vi "LDA_Analysis_2.vi"() -> (5 "Plug in titles":string[](array[string]), 7 "Plug in values":string[](array[string]))   [LabVIEW 2010]
uses:
  Controls/Save_Data.ctl
  Globals/LDA_meas_global_1.vi
  Globals/Plug_in_data_global.vi
  Globals/Meas_global.vi
  Globals/Constants_global.vi
  <vilib>/Analysis/NI_AALBase.lvlib
panel:
  out "Uneven timetrace":cluster{"Freq":dbl[], dbl[]}(graph)
  out "XY Graph 2":cluster{"Freq":dbl[], dbl[]}[](graph)
  in  "No of estimates output":i32=300
  out "Autocorrelation":cluster{dbl, dbl, dbl[]}[](graph)
  in  "Mode":enum16{"Spectra", "Autocorrelation"}(ring)
  in  "Separation Character":string="\t"
  in  "Precision":i16=2
  out "Ch names":string[](array[string])
  out "Number or Good blocks":i32
  out "Resampled block length":i32
  out "Resampling Frequency":dbl
  in  "Output Directory":path
  in  "File":T1=enum."Save Data"
  out "Frequency Spectrum":cluster{dbl, dbl, dbl[]}[](graph)
  # "You must have just these two indicators on the connector pane of the vi"
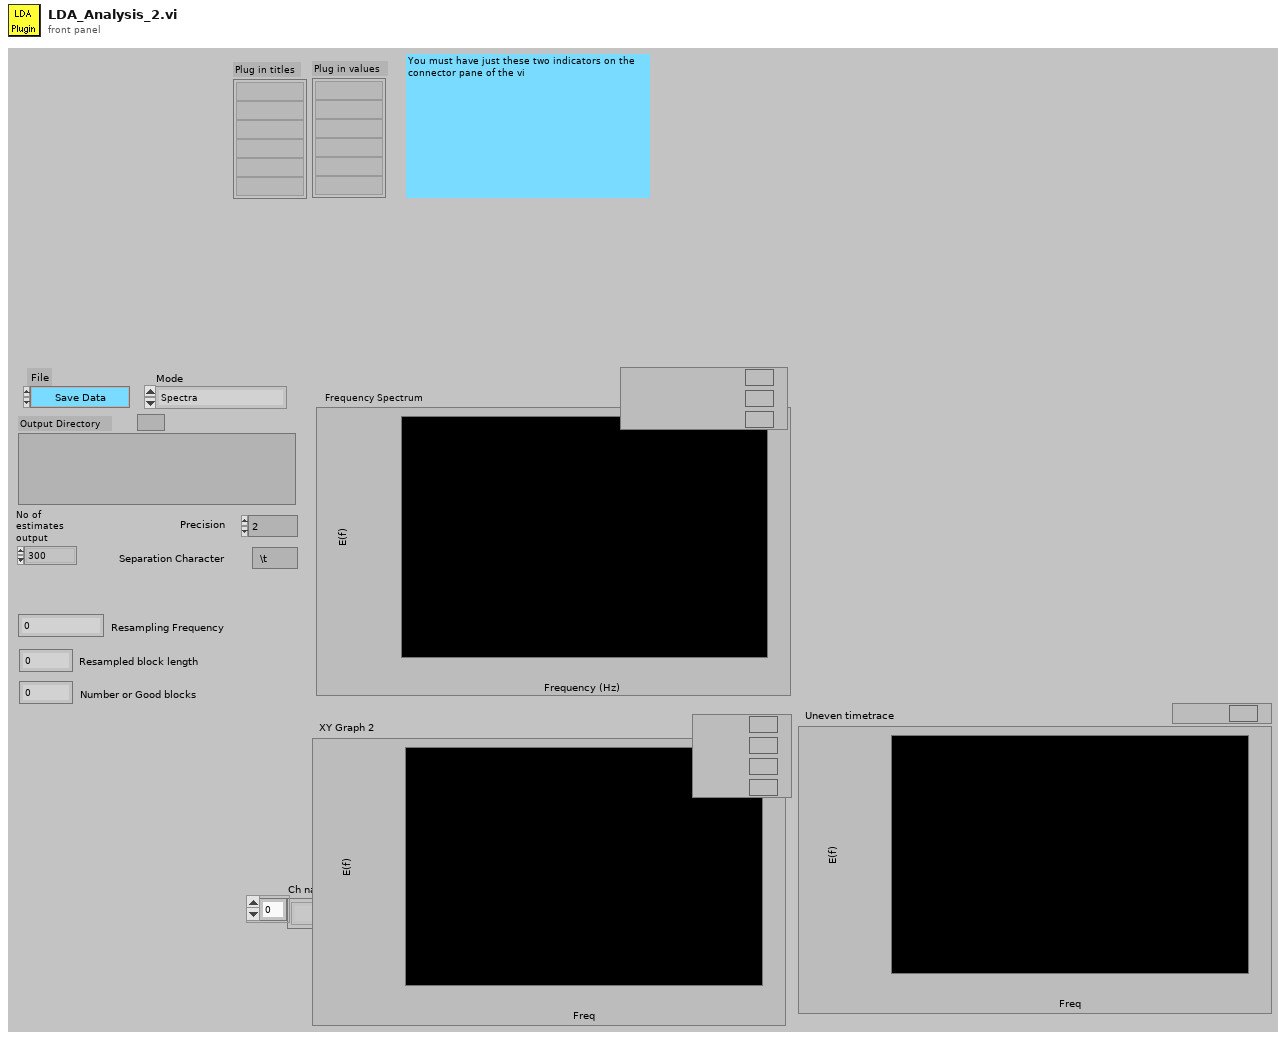
[diagram p1: front panel]
types:
  T1 = typedef "Save_Data.ctl" = enum16{"Save No Data", "Save Data"}
  T2 = enum32{"existing file", "new file", "new or existing file", "existing dir", "new dir", "new or existing dir", "existing file (use LLBs)", "new file (use LLBs)", "new or existing file (use LLBs)", "new or existing file or directory (use LLBs)"}
  T3 = typedef "Analysis_info_cluster.ctl" = cluster{"Colour":u32, "Inst type":T4, "Inst name":string, "Symbol":string, "Code name":string, "Extra Info":string, "Inst Array":T5, "Index":i32, "Voltage Index":i32, "Extra Titles":string[], "Extra Values":string[]}
  T4 = typedef "Inst_type.ctl" = enum16{"Propeller anemometer", "Raw voltage", "Pressure Transducer", "Pitot-static tube", "Preston tube", "Hot wire", "Cross wire 1", "Cross wire 2", "Generic Linear", "Generic Polynomial", "Generic BackPoly", "Fast FID", "Thermocouple", "Cold wire", "Pulsed Wire", "LDA Vel", "LDA Tran time", "LDA Arr time"}
  T5 = typedef "Instrument_Array.ctl" = enum16{"PWA", "LDA", "Analogue"}
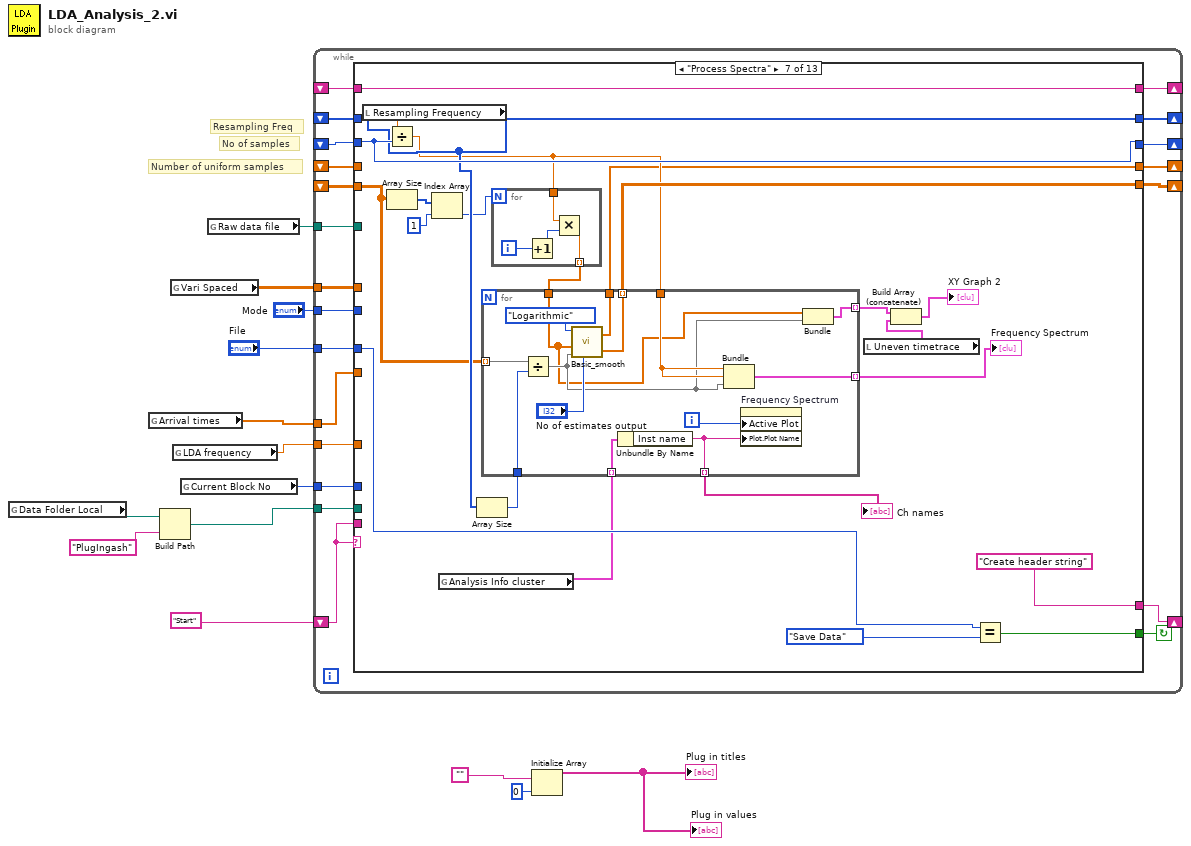
[diagram p0: block diagram]
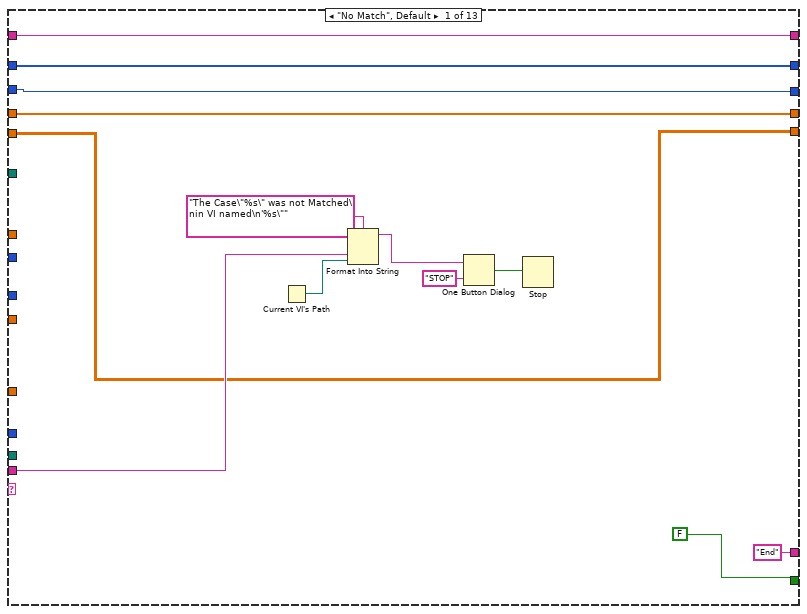
[diagram p2: hidden frame]
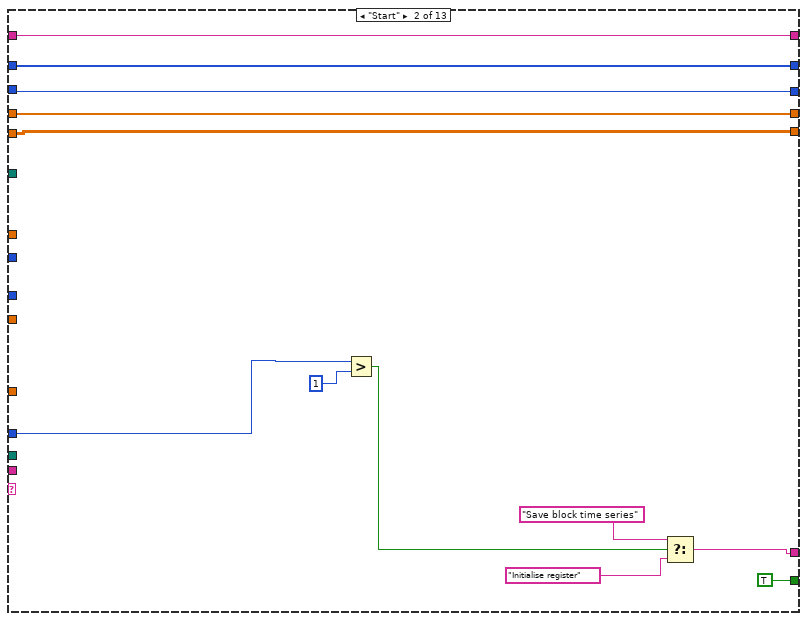
[diagram p3: hidden frame]
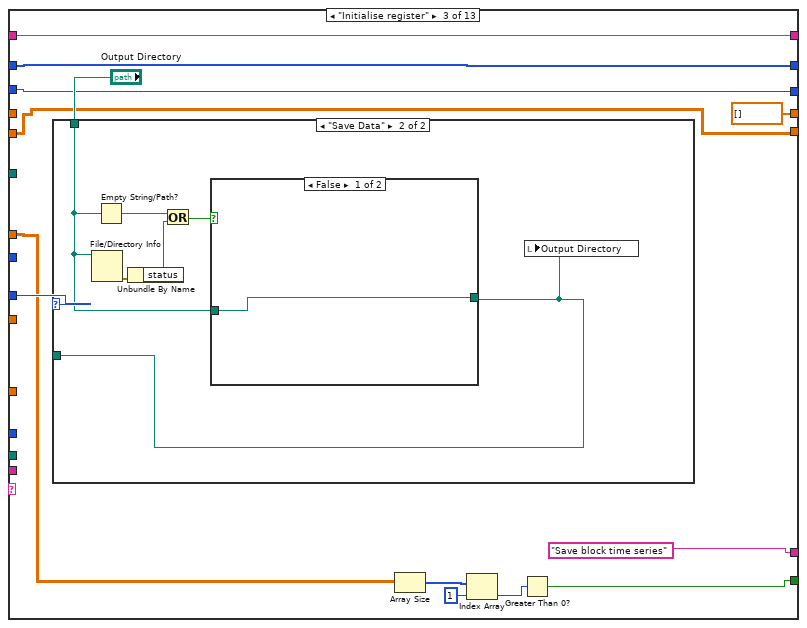
[diagram p4: hidden frame]
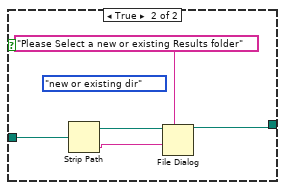
[diagram p6: hidden frame]
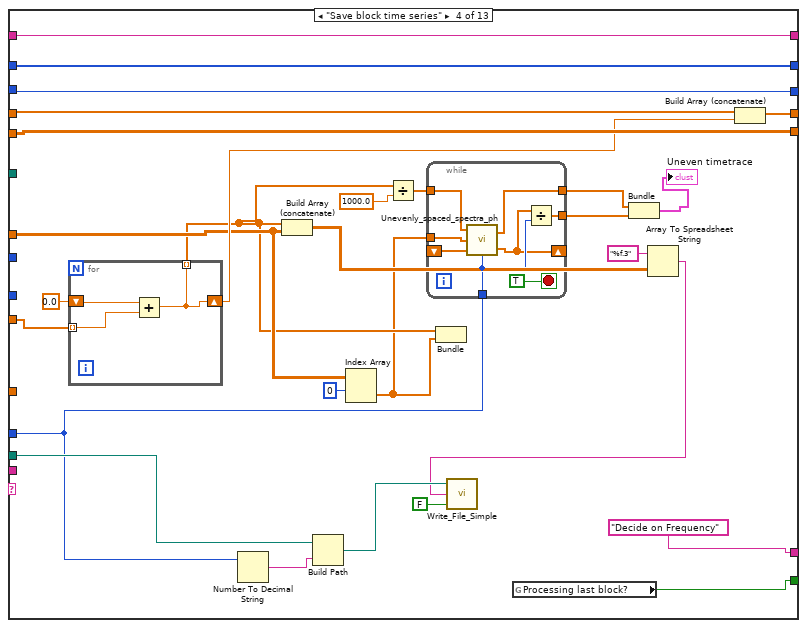
[diagram p7: hidden frame]
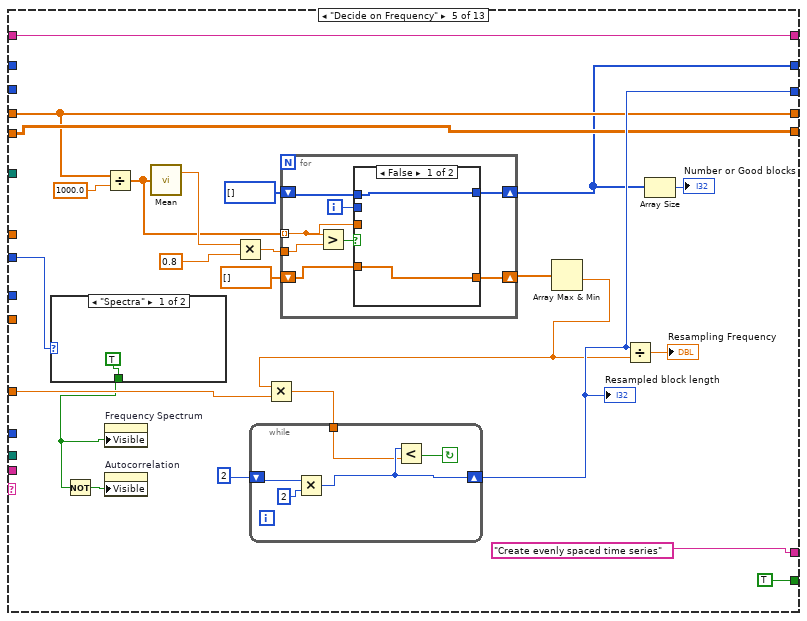
[diagram p8: hidden frame]
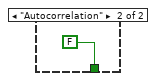
[diagram p9: hidden frame]
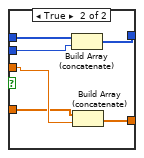
[diagram p10: hidden frame]
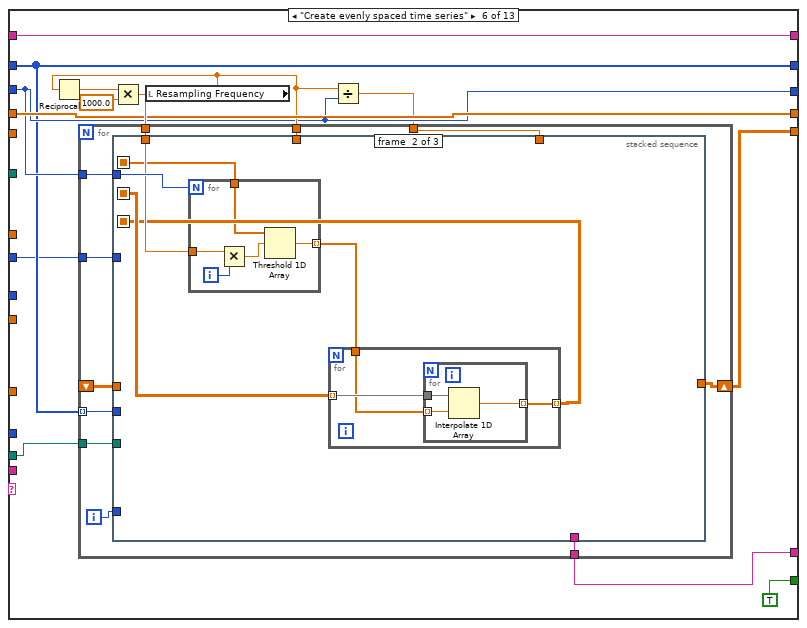
[diagram p11: hidden frame]
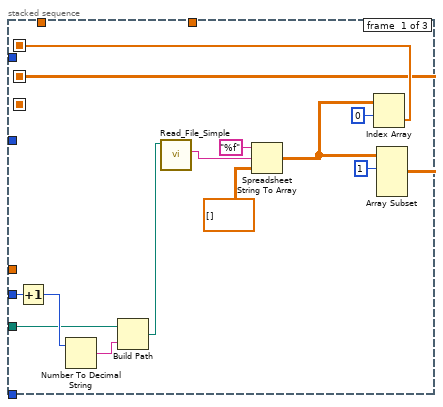
[diagram p12: hidden frame]
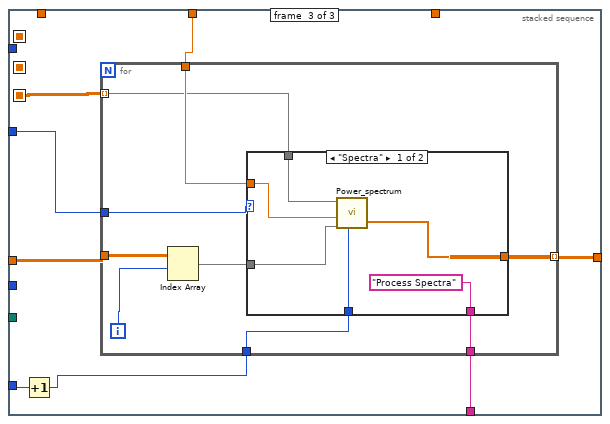
[diagram p13: hidden frame]
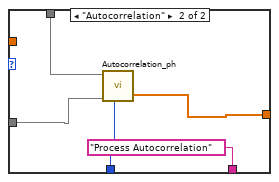
[diagram p14: hidden frame]
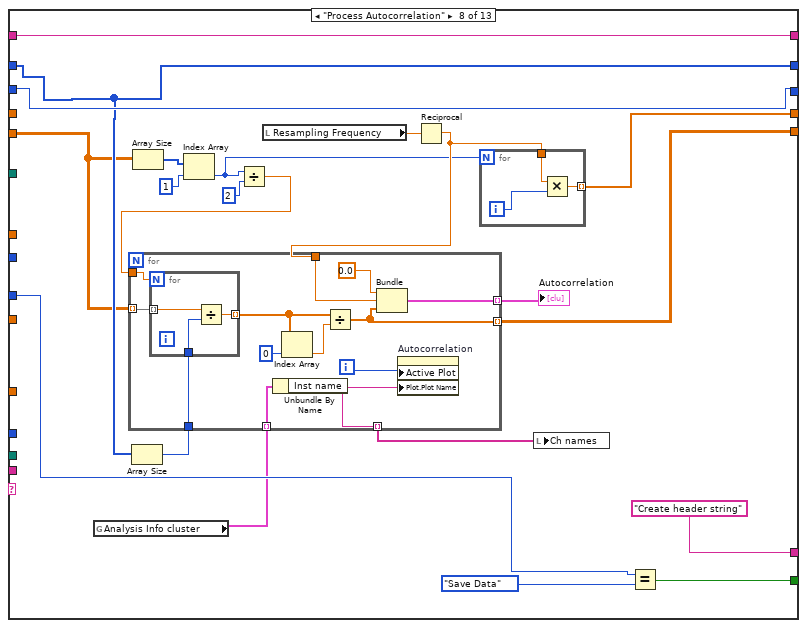
[diagram p15: hidden frame]
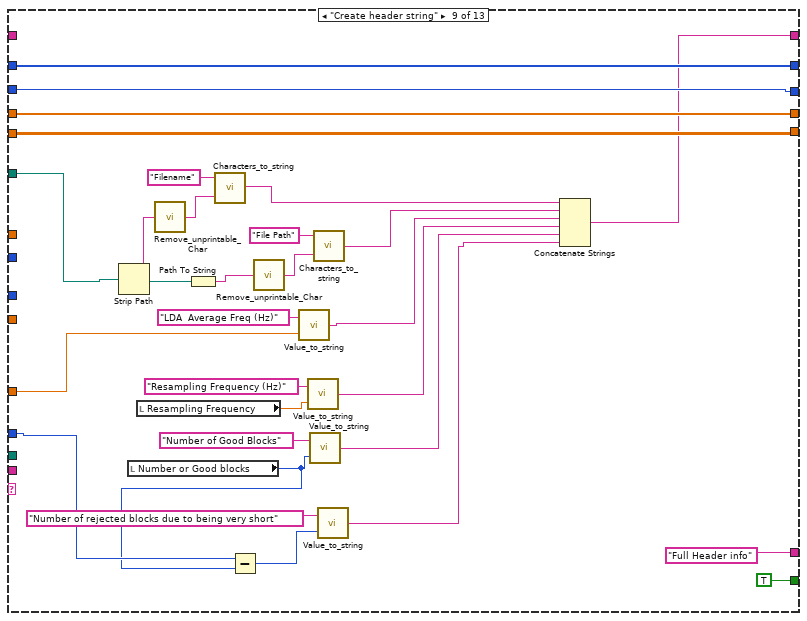
[diagram p16: hidden frame]
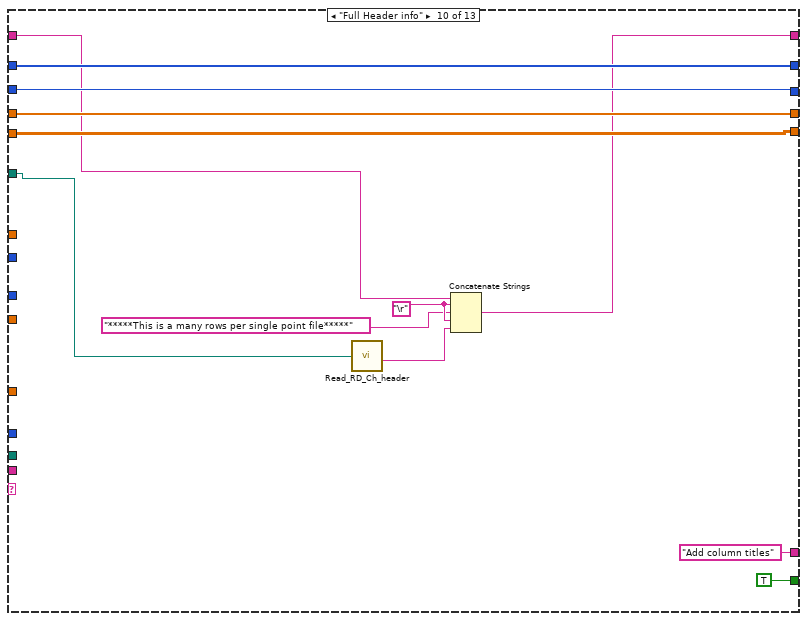
[diagram p17: hidden frame]
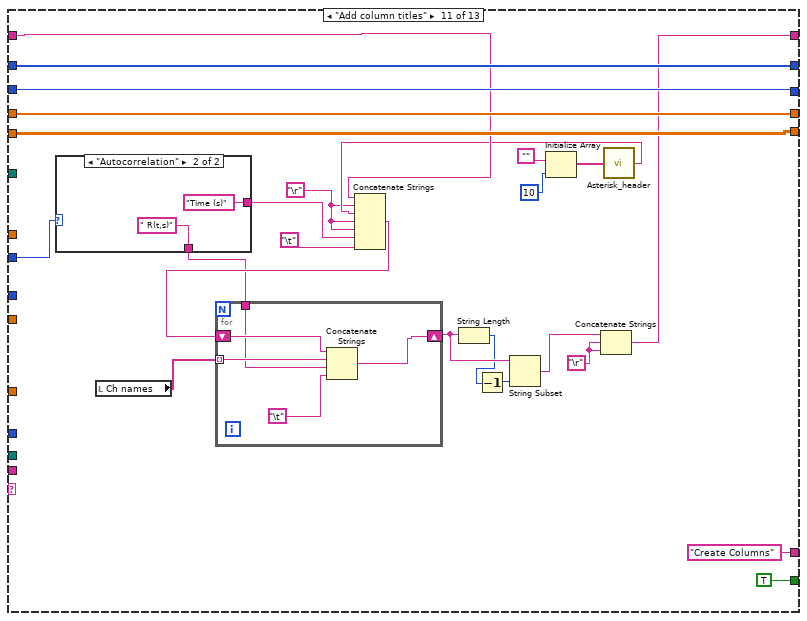
[diagram p18: hidden frame]
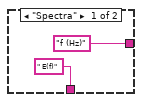
[diagram p19: hidden frame]
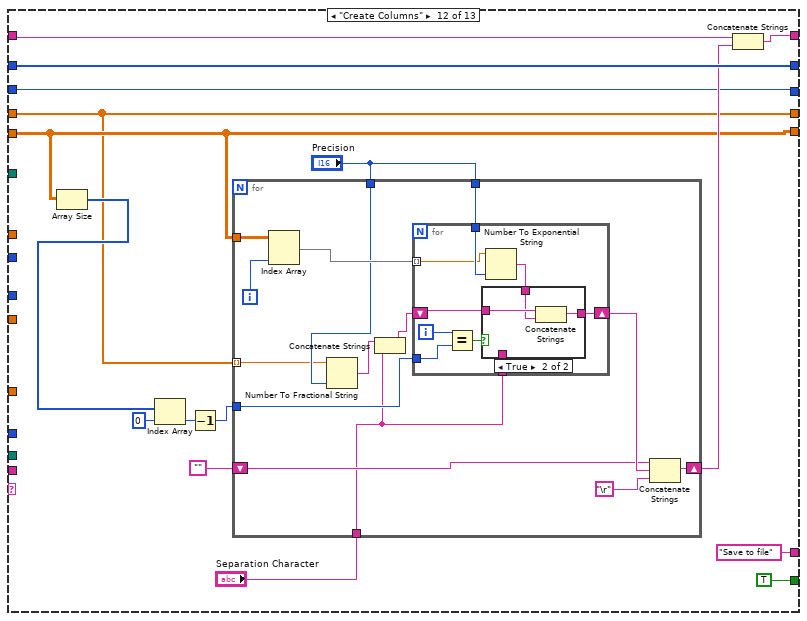
[diagram p20: hidden frame]
diagram:
  # "No of samples"
  # "Number of uniform samples"
  # "Resampling Freq"
  n1 = global read "Constants_global.vi" "Data Folder Local"() -> (w6:path)
  n2 = global read "LDA_meas_global_1.vi" "Arrival times"() -> (w12:dbl[])
  n3 = Build Path(base path=w6, name or relative path="PlugIngash") -> (appended path=w5:path)
  n4 = global read "Plug_in_data_global.vi" "Vari Spaced"() -> (w13:dbl[][])
  n5 = global read "Meas_global.vi" "LDA frequency"() -> (w2:dbl)
  n6 = global read "Meas_global.vi" "Current Block No"() -> (w8:i32)
  n7 = global read "Meas_global.vi" "Raw data file"() -> (w3:path)
  n8 = while {
    shift-left: "Start" -> [w35]
    shift-right: [w32] -> _
    tunnel: w13 -> [w34]
    tunnel: w12 -> [w33]
    shift-right: [w30] -> _
    shift-left: _ -> [w29]
    shift-right: [w28] -> _
    shift-left: _ -> [w27]
    tunnel: w8 -> [w26]
    tunnel: w5 -> [w25]
    shift-right: [w24] -> _
    shift-left: _ -> [w23]
    tunnel: "File" -> [w22]
    shift-right: [w21] -> _
    shift-left: _ -> [w20]
    tunnel: w3 -> [w19]
    tunnel: w2 -> [w18]
    shift-right: [w17] -> _
    shift-left: _ -> [w16]
    tunnel: "Mode" -> [w15]
    stop <- w31 continue-if-true
    n9 = case shown="\"Process Spectra\"" w35 {
      tunnel: ["End" ("t") w55 "Save block time series" ("t") "Decide on Frequency" ("t") "Create evenly spaced time series" ("t") w173 "Create header string" "Create header string" "Full Header info" ("t") "Add column titles" ("t") "Create Columns" ("t") "Save to file" ("t") "End" ("t")] -> w32
      tunnel: w35 -> [w44 _ _ _ _ _ _ _ _ _ _ _ _]
      tunnel: w34 -> [_ _ w65 w95 _ _ _ _ _ _ _ _ _]
      tunnel: w33 -> [_ _ _ w102 _ _ _ _ _ _ _ _ _]
      tunnel: [FALSE TRUE w61 w107 TRUE TRUE ("Processing last block?") w273 w313 TRUE ("Processing last block?") TRUE ("Processing last block?") TRUE ("Processing last block?") TRUE ("Processing last block?") FALSE] -> w31
      tunnel: [w41 w51 w68 w103 w142 w182 w269 w307 w340 w375 w399 w417 _] -> w30
      tunnel: w29 -> [w41 w51 w68 w103 w142 _ w261 w304 w340 w375 w399 w417 _]
      tunnel: [w39 w54 dbl[] [] w105 w138 w181 w264 w298 w341 w376 w400 w412 w471] -> w28
      tunnel: w27 -> [w39 w54 _ w106 w138 w181 _ _ w341 w376 w400 w412 w471]
      tunnel: w26 -> [_ w53 _ w90 _ _ _ _ w349 _ _ _ _]
      tunnel: w25 -> [_ _ _ w112 _ w184 _ _ _ _ _ _ _]
      tunnel: [w40 w52 w69 w104 w143 w178 w276 w316 w342 w377 w401 w419 w472] -> w24
      tunnel: w23 -> [w40 w52 w69 w104 _ w178 w276 w316 w342 w377 w401 w419 w472]
      tunnel: w22 -> [_ _ w70 _ _ _ w274 w314 _ _ _ _ _]
      tunnel: [w38 w50 w67 w99 w132 w176 w268 w310 w343 w378 w402 w427 w470] -> w21
      tunnel: w20 -> [w38 w50 w67 w99 _ w176 w268 w310 w343 w378 w402 w427 w470]
      tunnel: w19 -> [_ _ _ _ _ _ _ _ w355 w368 _ _ w469]
      tunnel: w18 -> [_ _ _ _ w130 _ _ _ w352 _ _ _ _]
      tunnel: [w37 w49 w66 w98 w129 w175 w272 w312 w339 w367 w395 w423 w461] -> w17
      tunnel: w16 -> [w37 w49 w66 w98 w129 w175 w272 w312 _ w374 w389 w424 w461]
      tunnel: w15 -> [_ _ _ _ w128 w174 _ _ _ _ w392 _ w458]
      frame "No Match", Default {
        n10 = Current VI's Path() -> (path=w43:path)
        n11 = Format Into String(format string="The Case\"%s\" was not Matched\nin VI named\n'%s\"" ("Format String"), w44, w43) -> (resulting string=w47:string)  [unwired: 2 in, 1 out]
        n12 = One Button Dialog(message=w47, button name ("OK")="STOP") -> (true=w45:bool)
        n13 = Stop(stop? (T)=w45) -> ()
      }
      frame "Start" {
        n14 = Greater?(x=w53, y=1) -> (0:w57:bool)
        n15 = Select(t="Save block time series", s=w57, f="Initialise register") -> (s? t:f=w55:string)
      }
      frame "Initialise register" {
        n16 = case shown="\"Save Data\"" w70 {
          tunnel: [w74 w80] -> _
          tunnel: "Output Directory" -> [w74 w78]
          frame "Save No Data" {
          }
          frame "Save Data" {
            n17 = File/Directory Info(path=w78) -> (error out=w79:errorcluster)  [unwired: 1 in, 6 out]
            n18 = Empty String/Path?(string/path=w78) -> (empty?=w76:bool)
            n19 = Unbundle By Name(w79) -> ("status"=w77:bool)
            n20 = Or(x=w76, y=w77) -> (x .or. y?=w75:bool)
            n21 = case shown="False" w75 {
              tunnel: [w81 w86] -> w80
              tunnel: w78 -> [w81 w84]
              frame False {
              }
              frame True {
                (unwired) T2."new or existing dir" ("select mode (2)")
                n22 = Strip Path(path=w84) -> (stripped path=w83:path, name=w82:string)
                n23 = File Dialog(7:"Please Select a new or existing Results folder" ("prompt"), 9:w82, 11:w83) -> (3:w86:path)  [unwired: 1 in, 6 out]
              }
            }
            n24 = local write "Output Directory"(w80) -> ()
          }
        }
        n25 = Array Size(array=w65) -> (size(s)=w64:i32[])
        n26 = Index Array(array=w64, index=1) -> (element=w62:i32)
        n27 = Greater Than 0?(x=w62) -> (x > 0?=w61:bool)
      }
      frame "Save block time series" {
        n28 = for {
          shift-right: [w123] -> w100
          shift-left: 0.0 -> [w125]
          tunnel: w102 -> [w124] mode=indexing
          tunnel: [w123] -> w94 mode=indexing
          n29 = Add(x=w125, y=w124) -> (x+y=w123:dbl)
        }
        n30 = Number To Decimal String(number=w90) -> (decimal integer string=w111:string)  [unwired: 1 out]
        n31 = Build Array (concatenate)(w94, w95) -> (w97:dbl[][])
        n32 = Build Path(base path=w112, name or relative path=w111) -> (appended path=w110:path)
        n33 = Index Array(array=w95, index (row)=0) -> (element=w91:dbl[])  [unwired: 1 in]
        n34 = Divide(x=w94, y=1000.0 ("x")) -> (x/y=w92:dbl[])
        n35 = while {
          tunnel: w92 -> [w122]
          tunnel: w91 -> [w121]
          shift-right: [w115] -> _
          shift-left: _ -> [w120]
          tunnel: w90 -> [w118]
          tunnel: [w119] -> w89
          tunnel: [w117] -> w88
          stop <- TRUE stop-if-true
          n36 = call "Unevenly_spaced_spectra_ph.vi"("Current Block No"=w118, "Shift in"=w120, "U"=w121, "Time"=w122) -> ("Sum E(F)"=w115:dbl[], "Freq"=w119:dbl[])
          n37 = Divide(x=w115, y=w118) -> (x/y=w117:dbl[])
        }
        n38 = Bundle(w94, "Vari Spaced"=w91) -> ()  [unwired: 1 in, 1 out]
        n39 = global read "Meas_global.vi" "Processing last block?"() -> (w107:bool)
        n40 = Bundle("Freq"=w89, w88) -> (→"Uneven timetrace":cluster{"Freq":dbl[], dbl[]})  [unwired: 1 in]
        n41 = Array To Spreadsheet String(array=w97, 3:"%f.3" ("format string")) -> (spreadsheet string=w109:string)  [unwired: 1 out]
        n42 = call "Write_File_Simple.vi"("append to file? (new file:F)"=FALSE, "character string"=w109, "file path"=w110) -> ()  [unwired: 2 out]
        n43 = Build Array (concatenate)(w106, w100) -> (w105:dbl[])
      }
      frame "Decide on Frequency" {
        n44 = case shown="\"Spectra\"" w128 {
          tunnel: [TRUE FALSE] -> w126
          frame "Spectra" {
          }
          frame "Autocorrelation" {
          }
        }
        n45 = Not(x=w126) -> (.not. x?=w127:bool)
        n46 = Divide(x=w138, y=1000.0) -> (x/y=w136:dbl[])
        n47 = property on="Frequency Spectrum" class="WFGraph (strict)"("Visible"=w126) -> ()  [unwired: 2 in, 2 out]
        n48 = property on="Autocorrelation" class="WFGraph (strict)"("Visible"=w127) -> ()  [unwired: 2 in, 2 out]
        n49 = call <vilib>:"Mean.vi"("X"=w136) -> ("mean"=w141:dbl)  [unwired: 1 out]
        n50 = Multiply(x=w141, y=0.8) -> (x*y=w139:dbl)
        n51 = for {
          tunnel: w136 -> [w154] mode=indexing
          tunnel: w139 -> [w159]
          shift-right: [w155] -> w132
          shift-left: i32[] [] -> [w156]
          shift-right: [w152] -> w134
          shift-left: dbl[] [] -> [w153]
          i -> [w157]
          n52 = Greater?(x=w154, y=w159) -> (0:w158:bool)
          n53 = case shown="False" w158 {
            tunnel: w157 -> [_ w167]
            tunnel: w156 -> [w161 w166]
            tunnel: [w161 w165] -> w155
            tunnel: w154 -> [_ w164]
            tunnel: w153 -> [w160 w163]
            tunnel: [w160 w162] -> w152
            frame False {
            }
            frame True {
              n54 = Build Array (concatenate)(w166, w167) -> (w165:i32[])
              n55 = Build Array (concatenate)(w163, w164) -> (w162:dbl[])
            }
          }
        }
        n56 = Array Max & Min(array=w134) -> (min value=w133:dbl)  [unwired: 3 out]
        n57 = Multiply(x=w133, y=w130) -> (x*y=w145:dbl)
        n58 = while {
          shift-right: [w170] -> w143
          shift-left: 2 -> [w172]
          tunnel: w145 -> [w169]
          stop <- w168 continue-if-true
          n59 = Multiply(x=w172, y=2) -> (x*y=w170:i32)
          n60 = Less?(x=w170, y=w169) -> (x < y?=w168:bool)
        }
        "Resampled block length" <- w143
        n61 = Divide(x=w143, y=w133) -> (x/y=→"Resampling Frequency":dbl)
        n62 = Array Size(array=w132) -> (size(s)=→"Number or Good blocks":i32)
      }
      frame "Create evenly spaced time series" {
        n63 = local read "Resampling Frequency"() -> (w179:dbl)
        n64 = Reciprocal(x=w179) -> (1/x=w185:dbl)
        n65 = Multiply(x=w185, y=1000.0) -> (x*y=w183:dbl)
        n66 = Divide(x=w179, y=w178) -> (x/y=w177:dbl)
        n67 = for {
          tunnel: w184 -> [w197]
          tunnel: w178 -> [w196]
          tunnel: w183 -> [w195]
          shift-right: [w193] -> w182
          shift-left: _ -> [w194]
          tunnel: w179 -> [w192]
          tunnel: w177 -> [w191]
          tunnel: w176 -> [w189] mode=indexing
          tunnel: w174 -> [w188]
          tunnel: [w187] -> w173
          i -> [w190]
          n68 = stacked-sequence {
            seq-local: [w203 _ _] -> [_ w214 _]
            seq-local: [w200 _ _] -> [_ w212 _]
            seq-local: [_ w211 _] -> [_ _ w235]
            tunnel: w190 -> [_ _ w231]
            tunnel: w197 -> [w208 _ _]
            tunnel: w196 -> [_ w216 _]
            tunnel: w195 -> [_ w215 _]
            tunnel: w194 -> [_ _ w234]
            tunnel: [_ _ w233] -> w193
            tunnel: w192 -> [_ _ w232]
            tunnel: w191 -> [_ _ _]
            tunnel: w189 -> [w198 _ _]
            tunnel: w188 -> [_ _ w229]
            tunnel: [_ _ w228] -> w187
            frame #0 {
              n69 = Increment(x=w198) -> (x+1=w209:i32)
              n70 = Number To Decimal String(number=w209) -> (decimal integer string=w210:string)  [unwired: 1 out]
              n71 = Build Path(base path=w208, name or relative path=w210) -> (appended path=w207:path)
              n72 = call "Read_File_Simple.vi"("Filename"=w207) -> ("string"=w206:string)  [unwired: 2 in, 7 out]
              n73 = Spreadsheet String To Array(format string="%f", spreadsheet string=w206, array type (2D Dbl)=dbl[][] []) -> (array=w202:dbl[][])  [unwired: 1 out]
              n74 = Index Array(array=w202, index (row)=0) -> (element=w203:dbl[])  [unwired: 1 in]
              n75 = Array Subset(array=w202, index (row)=1 ("index")) -> (w200:dbl[][])  [unwired: 3 in]
            }
            frame #1 {
              n76 = for {
                N: w216 -> [_]
                tunnel: w215 -> [w226]
                tunnel: w214 -> [w224]
                tunnel: [w223] -> w213 mode=indexing
                i -> [w227]
                n77 = Multiply(x=w226, y=w227) -> (x*y=w225:dbl)
                n78 = Threshold 1D Array(2:w225, 3:w224) -> (0:w223:dbl)  [unwired: 1 out]
              }
              n79 = for {
                tunnel: [w219] -> w211 mode=indexing
                tunnel: w213 -> [w217]
                tunnel: w212 -> [w218] mode=indexing
                n80 = for {
                  tunnel: w218 -> [w222]
                  tunnel: w217 -> [w221] mode=indexing
                  tunnel: [w220] -> w219 mode=indexing
                  n81 = Interpolate 1D Array(1:w221, 2:w222) -> (0:w220:dbl)
                }
              }
            }
            frame #2 {
              n82 = Increment(x=w231) -> (x+1=w230:i32)
              n83 = for {
                tunnel: w235 -> [w240] mode=indexing
                tunnel: [w239] -> w233 mode=indexing
                tunnel: w234 -> [w244]
                tunnel: w232 -> [w241]
                tunnel: w230 -> [w238]
                tunnel: w229 -> [w237]
                tunnel: [w236] -> w228
                i -> [w242]
                n84 = Index Array(array=w244, index (row)=w242) -> (element=w243:dbl[])  [unwired: 1 in]
                n85 = case shown="\"Spectra\"" w237 {
                  tunnel: w243 -> [w250 w254]
                  tunnel: w241 -> [w249 _]
                  tunnel: w240 -> [w248 w255]
                  tunnel: [w247 w253] -> w239
                  tunnel: w238 -> [w246 w252]
                  tunnel: ["Process Spectra" ("t") "Process Autocorrelation" ("t")] -> w236
                  frame "Spectra" {
                    n86 = call "Power_spectrum.vi"("U"=w248, "Sampling frequency"=w249, "Spectrum input array"=w250, "Block No"=w246) -> ("Spectrum output array"=w247:dbl[])  [unwired: 1 in, 1 out]
                  }
                  frame "Autocorrelation" {
                    n87 = call "Autocorrelation_ph.vi"("X"=w255, "Autocorrelation of X"=w254, "Block No"=w252) -> ("Autocorrelation of X"=w253:dbl[])  [unwired: 2 in, 1 out]
                  }
                }
              }
            }
          }
        }
      }
      frame "Process Spectra" {
        (unwired) FALSE
        n88 = local read "Resampling Frequency"() -> (w277:dbl)
        n89 = Divide(x=w277, y=w276) -> (x/y=w266:dbl)
        n90 = Array Size(array=w261) -> (size(s)=w263:i32[])
        n91 = Index Array(array=w263, index=1) -> (element=w260:i32)
        n92 = global read "Meas_global.vi" "Analysis Info cluster"() -> (w270:T3[])
        n93 = Array Size(array=w268) -> (size(s)=w267:i32)
        n94 = for {
          N: w260 -> [_]
          tunnel: w266 -> [w280]
          tunnel: [w279] -> w265 mode=indexing
          i -> [w282]
          n95 = Increment(x=w282) -> (x+1=w281:i32)
          n96 = Multiply(x=w280, y=w281) -> (x*y=w279:dbl)
        }
        n97 = for {
          tunnel: w266 -> [w296]
          tunnel: w261 -> [w295] mode=indexing
          tunnel: w267 -> [w294]
          tunnel: [w293] -> w259 mode=indexing
          tunnel: w270 -> [w291] mode=indexing
          tunnel: [w290] -> w271 mode=indexing
          tunnel: [w287] -> w269 mode=indexing
          tunnel: w265 -> [w284]
          tunnel: [w286] -> w264
          tunnel: [w283] -> w258 mode=indexing
          i -> [w292]
          n98 = Divide(x=w295, y=w294) -> (x/y=w285:dbl[])
          n99 = call "Basic_smooth.vi"("Smoothing"=enum16{"Linear", "Logarithmic"}."Logarithmic", "X array in"=w284, "Y array in"=w285, "No of estimates output"="No of estimates output") -> ("X array Out"=w286:dbl[], "Y array Out"=w287:dbl[])  [unwired: 1 out]
          n100 = Unbundle By Name(w291) -> ("Inst name"=w290:string)
          n101 = Bundle(w296, w296, w285) -> (w293:cluster{dbl, dbl, dbl[]})  [unwired: 1 out]
          n102 = property on="Frequency Spectrum" class="WFGraph (strict)"("Active Plot"=w292, "Plot.Plot Name"=w290) -> ()  [unwired: 2 in, 2 out]
          n103 = Bundle(w284, w285) -> (w283:cluster{dbl[], dbl[]})  [unwired: 1 in]
        }
        "Frequency Spectrum" <- w259
        "Ch names" <- w271
        n104 = local read "Uneven timetrace"() -> (w256:cluster{"Freq":dbl[], dbl[]})
        n105 = Build Array (concatenate)(w258, w256) -> (→"XY Graph 2":cluster{"Freq":dbl[], dbl[]}[])
        n106 = Equal?(x=w274, y=Save_Data."Save Data" ("File")) -> (x = y?=w273:bool)
      }
      frame "Process Autocorrelation" {
        (unwired) FALSE
        n107 = global read "Meas_global.vi" "Analysis Info cluster"() -> (w311:T3[])
        n108 = Array Size(array=w310) -> (size(s)=w309:i32)
        n109 = Array Size(array=w304) -> (size(s)=w303:i32[])
        n110 = Index Array(array=w303, index=1) -> (element=w297:i32)
        n111 = Divide(x=w297, y=2) -> (x/y=w300:dbl)
        n112 = local read "Resampling Frequency"() -> (w308:dbl)
        n113 = Reciprocal(x=w308) -> (1/x=w299:dbl)
        n114 = for {
          tunnel: w299 -> [w333]
          tunnel: w304 -> [w332] mode=indexing
          tunnel: w309 -> [w331]
          tunnel: [w330] -> w305 mode=indexing
          tunnel: w311 -> [w329] mode=indexing
          tunnel: [w324] -> w307 mode=indexing
          tunnel: [w322] -> w306 mode=indexing
          tunnel: w300 -> [w321]
          i -> [w323]
          n115 = for {
            N: w321 -> [_]
            tunnel: w332 -> [w336] mode=indexing
            tunnel: w331 -> [w335]
            tunnel: [w334] -> w326 mode=indexing
            n116 = Divide(x=w336, y=w335) -> (x/y=w334:dbl)
          }
          n117 = Unbundle By Name(w329) -> ("Inst name"=w322:string)
          n118 = Index Array(array=w326, index=0) -> (element=w325:dbl)
          n119 = Divide(x=w326, y=w325) -> (x/y=w324:dbl[])
          n120 = Bundle(0.0, w333, w324) -> (w330:cluster{dbl, dbl, dbl[]})  [unwired: 1 out]
          n121 = property on="Autocorrelation" class="WFGraph (strict)"("Active Plot"=w323, "Plot.Plot Name"=w322) -> ()  [unwired: 2 in, 2 out]
        }
        "Autocorrelation" <- w305
        n122 = for {
          N: w297 -> [_]
          tunnel: w299 -> [w320]
          tunnel: [w318] -> w298 mode=indexing
          i -> [w319]
          n123 = Multiply(x=w320, y=w319) -> (x*y=w318:dbl)
        }
        n124 = local write "Ch names"(w306) -> ()
        n125 = Equal?(x=w314, y=Save_Data."Save Data" ("File")) -> (x = y?=w313:bool)
      }
      frame "Create header string" {
        n126 = Strip Path(path=w355) -> (stripped path=w359:path, name=w363:string)
        n127 = local read "Number or Good blocks"() -> (w348:i32)
        n128 = local read "Resampling Frequency"() -> (w351:dbl)
        n129 = call "Remove_unprintable_Char.vi"("Input String"=w363) -> ("Output String"=w362:string)
        n130 = Path To String(path=w359) -> (string=w358:string)
        n131 = call "Characters_to_string.vi"("Characters to write"=w362, "Label for characters"="Filename") -> ("Output string"=w357:string)
        n132 = Subtract(x=w349, y=w348) -> (x-y=w347:i32)
        n133 = call "Remove_unprintable_Char.vi"("Input String"=w358) -> ("Output String"=w361:string)
        n134 = call "Value_to_string.vi"("Value"=w352, "Label for value"="LDA  Average Freq (Hz)") -> ("Output string"=w366:string)  [unwired: 1 in]
        n135 = call "Value_to_string.vi"("Value"=w351, "Label for value"="Resampling Frequency (Hz)") -> ("Output string"=w346:string)  [unwired: 1 in]
        n136 = call "Value_to_string.vi"("Value"=w348, "Label for value"="Number of Good Blocks") -> ("Output string"=w345:string)  [unwired: 1 in]
        n137 = call "Characters_to_string.vi"("Characters to write"=w361, "Label for characters"="File Path") -> ("Output string"=w356:string)
        n138 = call "Value_to_string.vi"("Value"=w347, "Label for value"="Number of rejected blocks due to being very short") -> ("Output string"=w344:string)  [unwired: 1 in]
        n139 = Concatenate Strings(w357, w356, w366, w346, w345, w344) -> (w339:string)
      }
      frame "Full Header info" {
        w371 = "\r"
        n140 = call "Read_RD_Ch_header.vi"("Raw data file"=w368) -> ("Ch string"=w369:string)  [unwired: 3 out]
        n141 = Concatenate Strings(w374, w371, "*****This is a many rows per single point file*****", w371, w369) -> (w367:string)
      }
      frame "Add column titles" {
        w383 = "\r"
        w384 = "\r"
        n142 = case shown="\"Autocorrelation\"" w392 {
          tunnel: ["f (Hz)" "Time (s)"] -> w391
          tunnel: [" E(f)" " R(t,s)"] -> w390
          frame "Spectra" {
          }
          frame "Autocorrelation" {
          }
        }
        n143 = local read "Ch names"() -> (w397:string[])
        n144 = Initialize Array("", 10) -> (w388:string[])
        n145 = call "Asterisk_header.vi"("Channel names"=w388) -> ("Header string"=w385:string)
        n146 = Concatenate Strings(w389, w383, w385, w383, w383, w391, "\t") -> (w396:string)
        n147 = for {
          shift-right: [w408] -> w382
          shift-left: w396 -> [w410]
          tunnel: w397 -> [w411] mode=indexing
          tunnel: w390 -> [w407]
          n148 = Concatenate Strings(w410, w411, w407, "\t") -> (w408:string)
        }
        n149 = String Length(string=w382) -> (length=w379:i32)
        n150 = Decrement(x=w379) -> (x-1=w380:i32)
        n151 = String Subset(string=w382, length (rest)=w380) -> (substring=w381:string)  [unwired: 1 out]
        n152 = Concatenate Strings(w381, w384, w384) -> (w395:string)
      }
      frame "Create Columns" {
        n153 = Array Size(array=w417) -> (size(s)=w415:i32[])
        n154 = Index Array(array=w415, index=0) -> (element=w414:i32)
        n155 = Decrement(x=w414) -> (x-1=w413:i32)
        n156 = for {
          shift-right: [w441] -> w422
          shift-left: "" -> [w436]
          tunnel: "Separation Character" -> [w429]
          tunnel: w417 -> [w439]
          tunnel: w413 -> [w435]
          tunnel: "Precision" -> [w433]
          tunnel: "Precision" -> [w432]
          tunnel: w412 -> [w428] mode=indexing
          i -> [w434]
          n157 = Index Array(array=w439, index (col)=w434) -> (element=w438:dbl[])  [unwired: 1 in]
          n158 = Number To Fractional String(number=w428, precision (6)=w432) -> (F-format string=w431:string)  [unwired: 2 out]
          n159 = Concatenate Strings(w431, w429) -> (w430:string)
          n160 = for {
            shift-right: [w448] -> w437
            shift-left: w430 -> [w450]
            tunnel: w429 -> [w447]
            tunnel: w438 -> [w442] mode=indexing
            tunnel: w435 -> [w445]
            tunnel: w433 -> [w443]
            i -> [w446]
            n161 = Equal?(x=w446, y=w445) -> (x = y?=w444:bool)
            n162 = Number To Exponential String(number=w442, precision (6)=w443) -> (E-format string=w449:string)  [unwired: 2 out]
            n163 = case shown="True" w444 {
              tunnel: w450 -> [w454 w457]
              tunnel: w449 -> [w453 w456]
              tunnel: [w452 w455] -> w448
              tunnel: w447 -> [w451 _]
              frame False {
                n164 = Concatenate Strings(w454, w453, w451) -> (w452:string)
              }
              frame True {
                n165 = Concatenate Strings(w457, w456) -> (w455:string)
              }
            }
          }
          n166 = Concatenate Strings(w436, w437, "\r") -> (w441:string)
        }
        n167 = Concatenate Strings(w424, w422) -> (w423:string)
      }
      frame "Save to file" {
        w463 = TRUE  # advisory dialog? (display:T)
        n168 = case shown="\"Autocorrelation\"" w458 {
          tunnel: ["Spec_" ("string") "Auto_" ("string")] -> w459
          frame "Spectra" {
          }
          frame "Autocorrelation" {
          }
        }
        n169 = Strip Path(path=w469) -> (name=w467:string)  [unwired: 1 out]
        n170 = local read "Output Directory"() -> (w468:path)
        n171 = Concatenate Strings(w459, w467) -> (w466:string)
        n172 = Build Path(base path=w468, name or relative path=w466) -> (appended path=w465:path)
        n173 = call "Create_directory_path.vi"("Path name"=w465) -> ("Path name Out"=w464:path)
        n174 = call "Write_Characters_To_File.vi"("file path (dialog if empty)"=w464, "advisory dialog? (display:T)"=w463, "character string"=w461, "append to file? (new file:F)"=FALSE) -> ()  [unwired: 1 in, 4 out]
      }
    }
  }
  n175 = Initialize Array("", 0) -> (→"Plug in values" →"Plug in titles":string[])
